vi "Read Lossless.vi"(0 "Depth (Unlimited)":i32=-1, 2 "EnclaveChannel":T2, 3 "timeout in ms (-1)":i32=-1) -> (7 "Element":T1, 8 "Closed?":bool, 9 "timed out?":bool)   [LabVIEW 2022 SP3, in "Enclave.lvlib"]
doc: "Reads data losslessly from the Channel Wire. <b>Depth</b> can be set on the first call of the endpoint to limit the number of elements that can be queued which will cause writers to block until space becomes available."
uses:
  Enclave.lvlib
  Lossless/Lossless.lvclass
  Element.ctl
  ))Channel.ctl
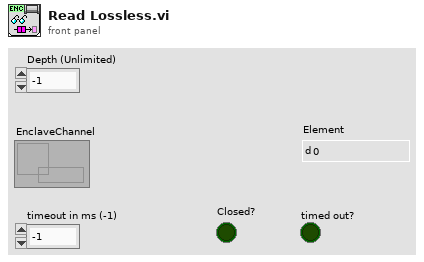
[diagram p1: front panel]
types:
  T1 = typedef "Enclave.lvlib/Element.ctl" = dbl
  T2 = typedef "Enclave.lvlib/))Channel.ctl" = refnum<queue>
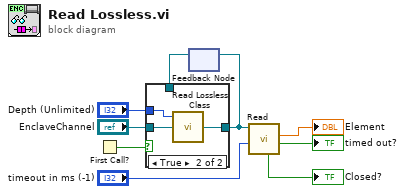
[diagram p0: block diagram]
diagram:
  n1 = First Call?() -> (First Call?: T/F=w9:bool)
  n2 = feedback #1() -> (w4:refnum<class "Lossless.lvclass">)  [unwired: 1 in]
  n3 = case shown="True" w9 {
    tunnel: "EnclaveChannel" -> [_ w13]
    tunnel: [w10 w12] -> w1
    tunnel: w4 -> [w10 _]
    tunnel: "Depth (Unlimited)" -> [_ w11]
    frame False {
    }
    frame True {
      n4 = call "Read Lossless Class.vi"("Depth (Unlimited)"=w11, "EnclaveChannel"=w13) -> ("Lossless"=w12:refnum<class "Lossless.lvclass">)  [unwired: 6 in, 1 out]
    }
  }
  n5 = feedback-in #1(w1) -> ()
  n6 = call "Read.vi"("timeout in ms (-1)"="timeout in ms (-1)", "Lossless in"=w1) -> ("timed out?"=→"timed out?":bool, "Element"=→"Element":T1, "Closed?"=→"Closed?":bool)  [unwired: 7 in]
